vi "Concatenating Tunnels.vi"() -> ()   [LabVIEW 2020]
uses:
  <vilib>/measure/NI_MABase.lvlib
panel:
  out "Waveform Graph - Indexing":dbl[][](graph)
  out "Waveform Graph - Concatenating":dbl[](graph)
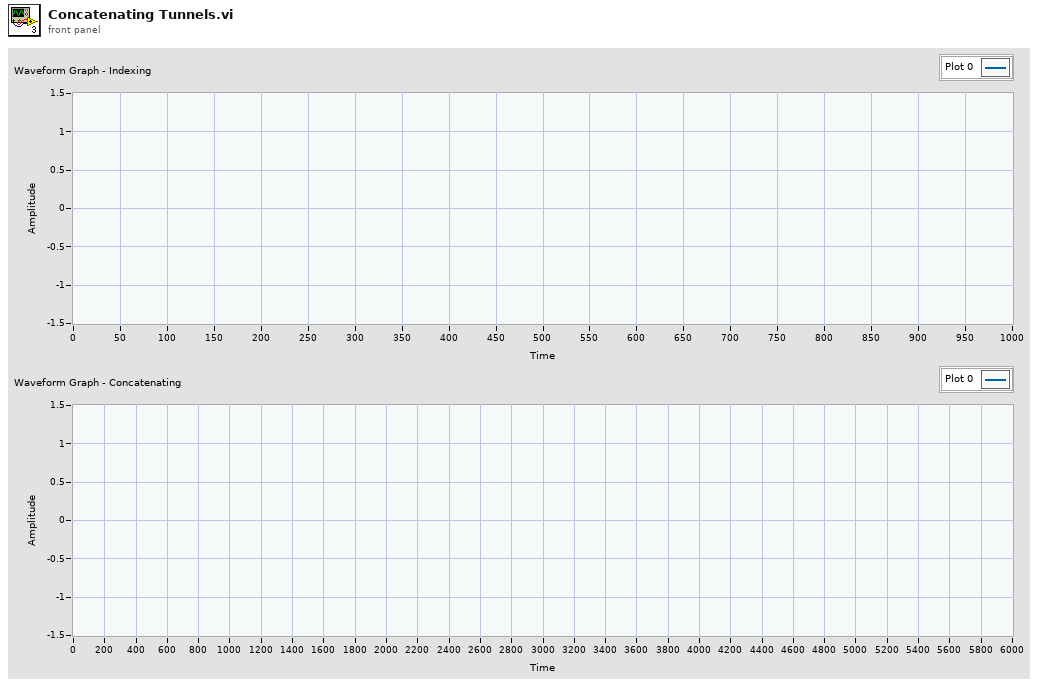
[diagram p1: front panel]
types:
  T1 = enum16{"Sine Wave", "Triangle Wave", "Square Wave", "Sawtooth Wave"}[]
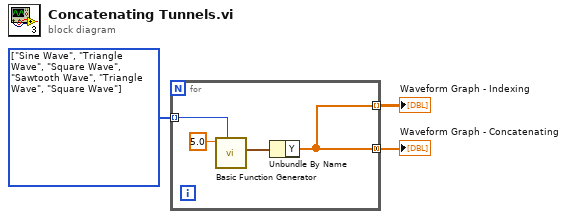
[diagram p0: block diagram]
diagram:
  w3 = T1 [enum."Sine Wave", enum."Triangle Wave", enum."Square Wave", enum."Sawtooth Wave", enum."Triangle Wave", enum."Square Wave"] items=["Sine Wave", "Triangle Wave", "Square Wave", "Sawtooth Wave"] ("signal type")
  n1 = for {
    tunnel: w3 -> [w7] mode=indexing
    tunnel: [w4] -> w2 mode=indexing
    tunnel: [w4] -> w1 mode=concatenating
    n2 = call <vilib>:"Basic Function Generator.vi"("signal type"=w7, "frequency"=5.0) -> ("signal out"=w6:waveform(dbl))  [unwired: 7 in, 2 out]
    n3 = Unbundle By Name(w6) -> ("Y"=w4:dbl[])
  }
  "Waveform Graph - Concatenating" <- w1
  "Waveform Graph - Indexing" <- w2
